vi "Alltesta Send.vi"(8 "error in (no error)":errorcluster, 10 "Command":string, 11 "Serial Port in":refnum<visa-resource-name>="COM3") -> (0 "error out":errorcluster, 2 "Response":string, 3 "Serial Port out":refnum<visa-resource-name>="COM3")   [LabVIEW 2023, in "Alltesta Autosampler.lvlib"]
uses:
  Alltesta Autosampler.lvlib
  <vilib>/Utility/error.llb/Trim Whitespace One-Sided.vi
panel:
  out "raw response":string
  out "Sent to device":string
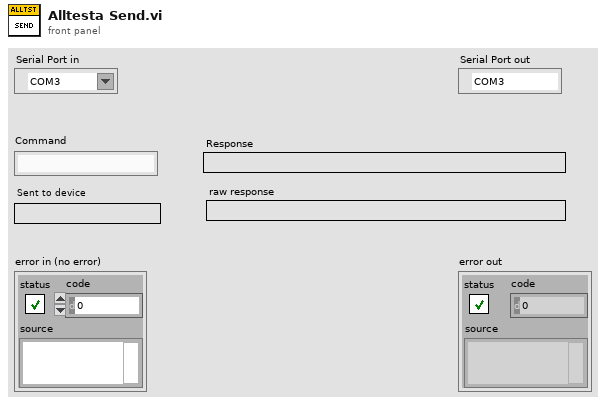
[diagram p1: front panel]
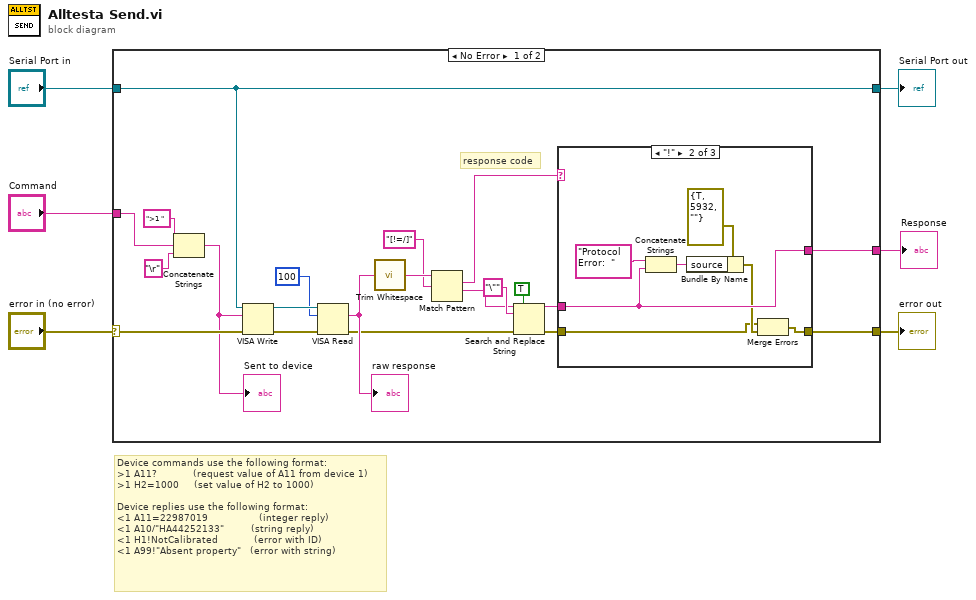
[diagram p0: block diagram]
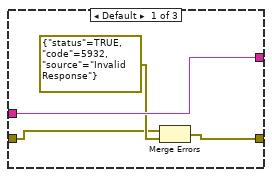
[diagram p2: hidden frame]
diagram:
  # "Device commands use the following format:\n>1 A11?            (request value of A11 from device 1)\n>1 H2=1000     (set value of H2 to 1000) \n\nDevice replies use the following format:\n<1 A11=22987019                 (integer reply)\n<1 A10/\"HA44252133\"         (string reply)\n<1 H1!NotCalibrated            (error with ID)\n<1 A99!\"Absent property\"   (error with string)"
  n1 = case shown="No Error" "error in (no error)" {
    selector: "error in (no error)" -> [w25 w41]
    tunnel: [w16 w41] -> w6
    tunnel: "Serial Port in" -> [w22 w40]
    tunnel: "Command" -> [w14 _]
    tunnel: [w22 w40] -> w2
    tunnel: [w15 _] -> w1
    frame No Error {
      # "response code"
      n2 = Concatenate Strings(">1 " ("string"), w14, "\r" ("string")) -> (w20:string)
      "Sent to device" <- w20
      n3 = VISA Write(VISA resource name=w22, write buffer=w20, error in (no error)=w25) -> (VISA resource name out=w24:refnum<visa-resource-name>, error out=w26:errorcluster)  [unwired: 1 out]
      n4 = VISA Read(VISA resource name=w24, byte count=u32 100, error in (no error)=w26) -> (read buffer=w19:string, error out=w17:errorcluster)  [unwired: 2 out]
      "raw response" <- w19
      n5 = call <vilib>:"Trim Whitespace.vi"("string"=w19) -> ("trimmed string"=w18:string)  [unwired: 1 in]
      n6 = Match Pattern(string=w18, regular expression="[!=/]") -> (match substring=w10:string, after substring=w9:string)  [unwired: 1 in, 2 out]
      n7 = Search and Replace String(replace all?=TRUE ("replace all? (F)"), input string=w9, search string="\"") -> (result string=w11:string)  [unwired: 5 in, 3 out]
      n8 = case shown="\"!\"" w10 {
        tunnel: w17 -> [w27 w31 w39]
        tunnel: [w30 w37 w39] -> w16
        tunnel: w11 -> [w29 w33 w38]
        tunnel: [w29 w33 w38] -> w15
        frame Default {
          n9 = Merge Errors(w27, errorcluster {"status"=TRUE, "code"=5932, "source"="Invalid Response"} ("error constant")) -> (w30:errorcluster)
        }
        frame "!" {
          n10 = Concatenate Strings("Protocol Error:  " ("string"), w33) -> (w35:string)
          n11 = Bundle By Name(cluster=errorcluster {"status"=TRUE, "code"=5932, "source"=""} ("error constant"), "source"=w35) -> (w32:errorcluster)
          n12 = Merge Errors(w31, w32) -> (w37:errorcluster)
        }
        frame "/", "=" {
          # "normal response"
        }
      }
    }
    frame Error {
    }
  }
  "error out" <- w6
  "Serial Port out" <- w2
  "Response" <- w1
